vi "labToString.vi"(11 "lab":dbl) -> (3 "String":string)   [LabVIEW 2014]
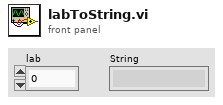
[diagram p1: front panel]
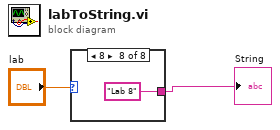
[diagram p0: block diagram]
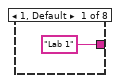
[diagram p2: hidden frame]
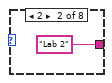
[diagram p3: hidden frame]
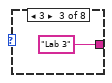
[diagram p4: hidden frame]
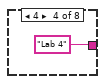
[diagram p5: hidden frame]
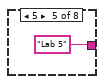
[diagram p6: hidden frame]
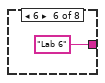
[diagram p7: hidden frame]
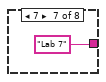
[diagram p8: hidden frame]
diagram:
  n1 = case shown="8" "lab" {
    tunnel: ["Lab 1" "Lab 2" "Lab 3" "Lab 4" "Lab 5" "Lab 6" "Lab 7" "Lab 8"] -> w2
    frame 1, Default {
    }
    frame 2 {
    }
    frame 3 {
    }
    frame 4 {
    }
    frame 5 {
    }
    frame 6 {
    }
    frame 7 {
    }
    frame 8 {
    }
  }
  "String" <- w2
